vi "parse rest of message.vi"(5 "timeout/kb ms (1)":i32=1, 7 "continuation timeout ms (2000)":i32=2000, 8 "error in":errorcluster, 10 "mask(1)+length(7)":u8, 11 "lvlibretls connection in":refnum<data-value>) -> (0 "error out":errorcluster, 3 "unmasked data":string)   [LabVIEW 2016, in "websocket core.lvlib"]
uses:
  websocket core.lvlib
  lvlibtls/socket connection/lvlibretls connection.lvclass
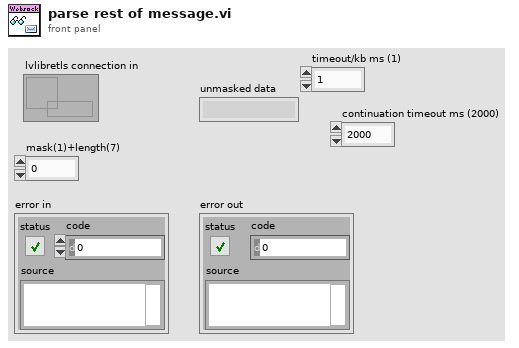
[diagram p1: front panel]
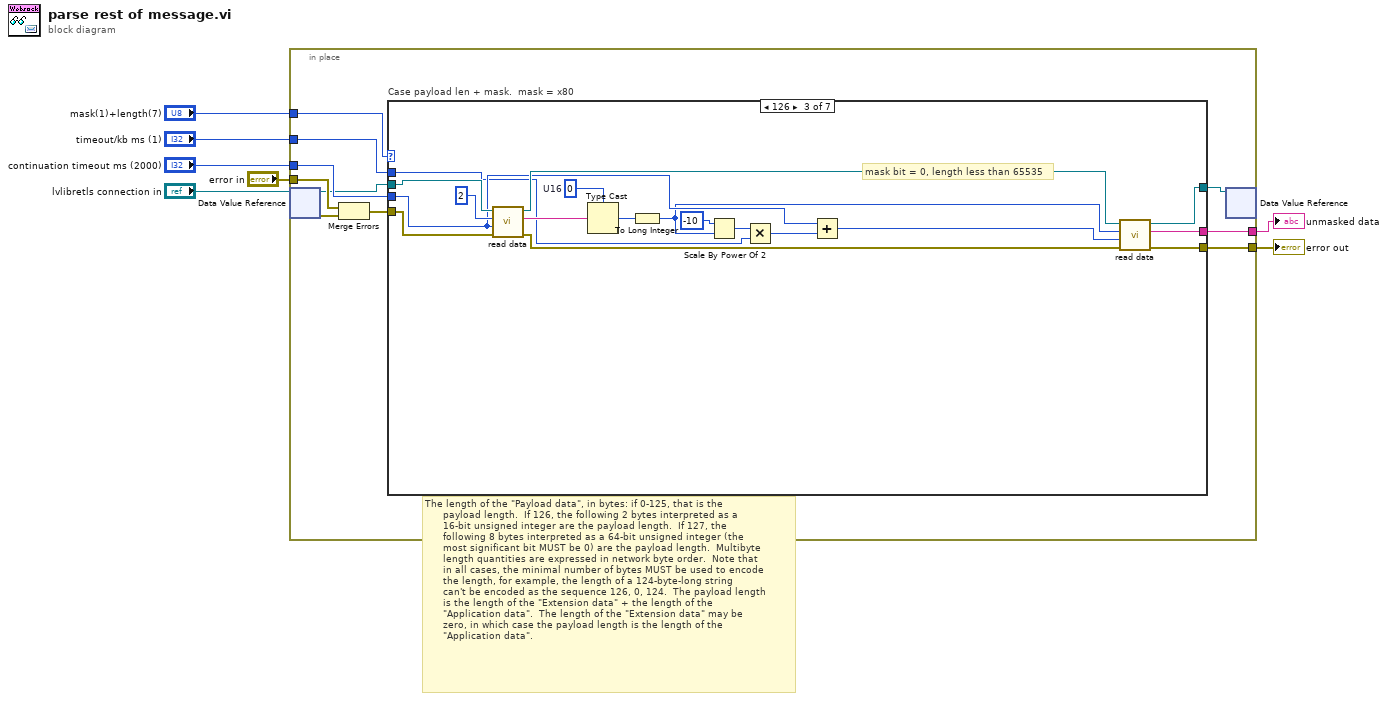
[diagram p0: block diagram]
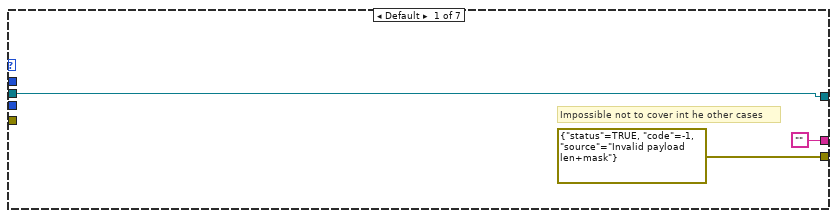
[diagram p2: hidden frame]
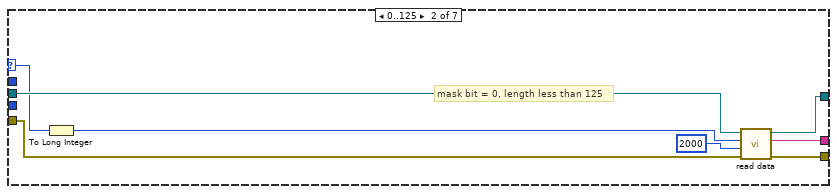
[diagram p3: hidden frame]
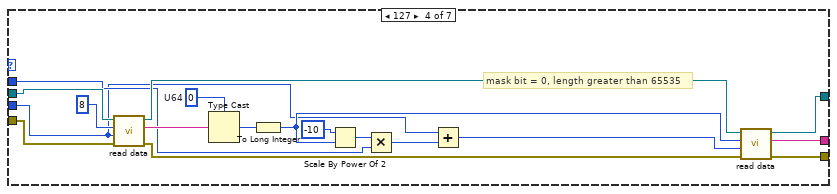
[diagram p4: hidden frame]
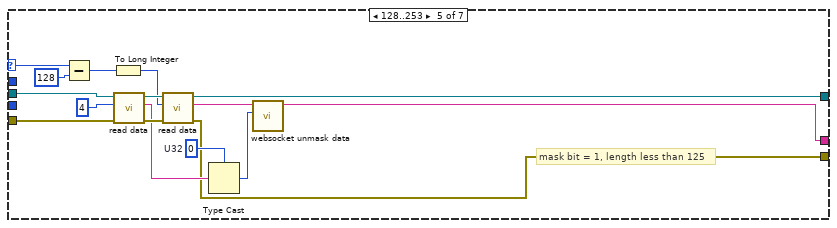
[diagram p5: hidden frame]
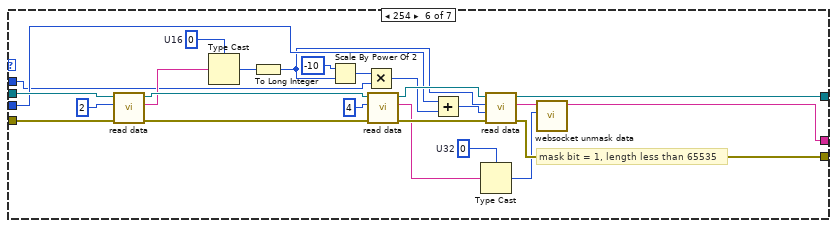
[diagram p6: hidden frame]
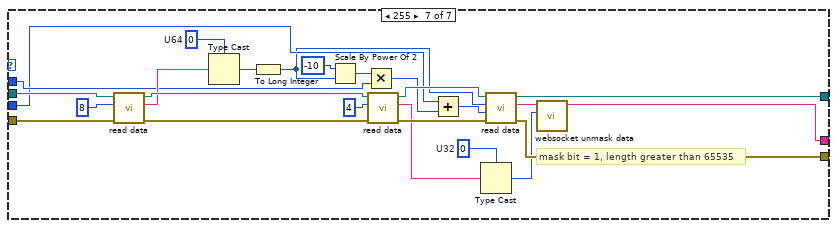
[diagram p7: hidden frame]
diagram:
  n1 = in-place {
    in-place-border: [w17] -> w7
    in-place-border: [w16] -> w6
    in-place-border: "mask(1)+length(7)" -> [w15]
    in-place-border: "error in" -> [w14]
    in-place-border: "continuation timeout ms (2000)" -> [w13]
    in-place-border: "timeout/kb ms (1)" -> [w12]
    # "The length of the \"Payload data\", in bytes: if 0-125, that is the\n      payload length.  If 126, the following 2 bytes interpreted as a\n      16-bit unsigned integer are the payload length.  If 127, the\n      following 8 bytes interpreted as a 64-bit unsigned integer (the\n      most significant bit MUST be 0) are the payload length.  Multibyte\n      length quantities are expressed in network byte order.  Note that\n      in all cases, the minimal number of bytes MUST be used to encode\n      the length, for example, the length of a 124-byte-long string\n      can't be encoded as the sequence 126, 0, 124.  The payload length\n      is the length of the \"Extension data\" + the length of the\n      \"Application data\".  The length of the \"Extension data\" may be\n      zero, in which case the payload length is the length of the\n      \"Application data\"."
    n2 = in-place-dvr #1("lvlibretls connection in") -> (w11:refnum<class "lvlibretls connection.lvclass">, w8:errorcluster)
    n3 = Merge Errors(w14, w8) -> (w9:errorcluster)
    n4 = case "Case payload len + mask.  mask = x80" shown="126" w15 {
      selector: w15 -> [_ w27 _ _ w79 _ _]
      tunnel: ["" w24 w39 w57 w68 w90 w115] -> w17
      tunnel: w11 -> [w18 w28 w46 w64 w80 w105 w130]
      tunnel: [errorcluster {"status"=TRUE, "code"=-1, "source"="Invalid payload len+mask"} ("error out") w23 w38 w56 w66 w94 w120] -> w16
      tunnel: w9 -> [_ w22 w37 w55 w70 w91 w116]
      tunnel: w13 -> [_ _ w36 w48 _ w85 w109]
      tunnel: w12 -> [_ _ w32 w49 _ w84 w110]
      tunnel: [w18 w21 w29 w47 w65 w81 w106] -> w10
      frame Default {
        # "Impossible not to cover int he other cases"
      }
      frame 0..125 {
        # "mask bit = 0, length less than 125"
        n5 = To Long Integer(number=w27) -> (32bit integer=w25:i32)
        n6 = call "read data.vi"("error in"=w22, "timeout"=2000 ("timeout ms (25000)"), "max size"=w25, "lvlibretls connection in"=w28) -> ("error out"=w23:errorcluster, "data"=w24:string, "lvlibretls connection out"=w21:refnum<class "lvlibretls connection.lvclass">)  [unwired: 5 in]
      }
      frame 126 {
        w40 = u16 0  # U16
        # "mask bit = 0, length less than 65535"
        n7 = call "read data.vi"("error in"=w37, "timeout"=w36, "max size"=2 ("bytes to read"), "lvlibretls connection in"=w46) -> ("error out"=w43:errorcluster, "data"=w42:string, "lvlibretls connection out"=w44:refnum<class "lvlibretls connection.lvclass">)  [unwired: 5 in]
        n8 = Type Cast(type=w40, x=w42) -> (*(type *) &x=w41:u16)
        n9 = To Long Integer(number=w41) -> (32bit integer=w35:i32)
        n10 = Scale By Power Of 2(n=i16 -10, x=w35) -> (x*2^n=w33:i32)
        n11 = Multiply(x=w33, y=w32) -> (x*y=w31:i32)
        n12 = Add(x=w36, y=w31) -> (x+y=w30:i32)
        n13 = call "read data.vi"("error in"=w43, "timeout"=w30, "max size"=w35, "lvlibretls connection in"=w44) -> ("error out"=w38:errorcluster, "data"=w39:string, "lvlibretls connection out"=w29:refnum<class "lvlibretls connection.lvclass">)  [unwired: 5 in]
      }
      frame 127 {
        w58 = u64 0  # U64
        # "mask bit = 0, length greater than 65535"
        n14 = call "read data.vi"("error in"=w55, "timeout"=w48, "max size"=8 ("bytes to read"), "lvlibretls connection in"=w64) -> ("error out"=w61:errorcluster, "data"=w60:string, "lvlibretls connection out"=w62:refnum<class "lvlibretls connection.lvclass">)  [unwired: 5 in]
        n15 = Type Cast(type=w58, x=w60) -> (*(type *) &x=w59:u64)
        n16 = To Long Integer(number=w59) -> (32bit integer=w51:i32)
        n17 = Scale By Power Of 2(n=i16 -10, x=w51) -> (x*2^n=w53:i32)
        n18 = Multiply(x=w53, y=w49) -> (x*y=w52:i32)
        n19 = Add(x=w48, y=w52) -> (x+y=w50:i32)
        n20 = call "read data.vi"("error in"=w61, "timeout"=w50, "max size"=w51, "lvlibretls connection in"=w62) -> ("error out"=w56:errorcluster, "data"=w57:string, "lvlibretls connection out"=w47:refnum<class "lvlibretls connection.lvclass">)  [unwired: 5 in]
      }
      frame 128..253 {
        w71 = u32 0  # U32
        # "mask bit = 1, length less than 125"
        n21 = Subtract(x=w79, y=u8 128) -> (x-y=w74:u8)
        n22 = To Long Integer(number=w74) -> (32bit integer=w73:i32)
        n23 = call "read data.vi"("error in"=w70, "max size"=4 ("bytes to read"), "lvlibretls connection in"=w80) -> ("error out"=w75:errorcluster, "data"=w72:string, "lvlibretls connection out"=w76:refnum<class "lvlibretls connection.lvclass">)  [unwired: 6 in]
        n24 = call "read data.vi"("error in"=w75, "max size"=w73, "lvlibretls connection in"=w76) -> ("error out"=w66:errorcluster, "data"=w69:string, "lvlibretls connection out"=w65:refnum<class "lvlibretls connection.lvclass">)  [unwired: 6 in]
        n25 = Type Cast(type=w71, x=w72) -> (*(type *) &x=w67:u32)
        n26 = call "websocket unmask data.vi"("mask key"=w67, "masked data"=w69) -> ("unmasked data"=w68:string)  [unwired: 9 in]
      }
      frame 254 {
        w92 = u32 0  # U32
        w99 = u16 0  # U16
        # "mask bit = 1, length less than 65535"
        n27 = call "read data.vi"("error in"=w91, "max size"=2 ("bytes to read"), "lvlibretls connection in"=w105) -> ("error out"=w102:errorcluster, "data"=w96:string, "lvlibretls connection out"=w103:refnum<class "lvlibretls connection.lvclass">)  [unwired: 6 in]
        n28 = Type Cast(type=w99, x=w96) -> (*(type *) &x=w100:u16)
        n29 = To Long Integer(number=w100) -> (32bit integer=w82:i32)
        n30 = Scale By Power Of 2(n=i16 -10, x=w82) -> (x*2^n=w87:i32)
        n31 = Multiply(x=w87, y=w84) -> (x*y=w86:i32)
        n32 = call "read data.vi"("error in"=w102, "max size"=4 ("bytes to read"), "lvlibretls connection in"=w103) -> ("error out"=w97:errorcluster, "data"=w93:string, "lvlibretls connection out"=w98:refnum<class "lvlibretls connection.lvclass">)  [unwired: 6 in]
        n33 = Add(x=w85, y=w86) -> (x+y=w83:i32)
        n34 = Type Cast(type=w92, x=w93) -> (*(type *) &x=w89:u32)
        n35 = call "read data.vi"("error in"=w97, "timeout"=w83, "max size"=w82, "lvlibretls connection in"=w98) -> ("error out"=w94:errorcluster, "data"=w95:string, "lvlibretls connection out"=w81:refnum<class "lvlibretls connection.lvclass">)  [unwired: 5 in]
        n36 = call "websocket unmask data.vi"("mask key"=w89, "masked data"=w95) -> ("unmasked data"=w90:string)  [unwired: 9 in]
      }
      frame 255 {
        w117 = u32 0  # U32
        w124 = u64 0  # U64
        # "mask bit = 1, length greater than 65535"
        n37 = call "read data.vi"("error in"=w116, "max size"=8 ("bytes to read"), "lvlibretls connection in"=w130) -> ("error out"=w127:errorcluster, "data"=w121:string, "lvlibretls connection out"=w128:refnum<class "lvlibretls connection.lvclass">)  [unwired: 6 in]
        n38 = Type Cast(type=w124, x=w121) -> (*(type *) &x=w125:u64)
        n39 = To Long Integer(number=w125) -> (32bit integer=w108:i32)
        n40 = Scale By Power Of 2(n=i16 -10, x=w108) -> (x*2^n=w112:i32)
        n41 = Multiply(x=w112, y=w110) -> (x*y=w111:i32)
        n42 = call "read data.vi"("error in"=w127, "max size"=4 ("bytes to read"), "lvlibretls connection in"=w128) -> ("error out"=w122:errorcluster, "data"=w118:string, "lvlibretls connection out"=w123:refnum<class "lvlibretls connection.lvclass">)  [unwired: 6 in]
        n43 = Add(x=w109, y=w111) -> (x+y=w107:i32)
        n44 = Type Cast(type=w117, x=w118) -> (*(type *) &x=w114:u32)
        n45 = call "read data.vi"("error in"=w122, "timeout"=w107, "max size"=w108, "lvlibretls connection in"=w123) -> ("error out"=w120:errorcluster, "data"=w119:string, "lvlibretls connection out"=w106:refnum<class "lvlibretls connection.lvclass">)  [unwired: 5 in]
        n46 = call "websocket unmask data.vi"("mask key"=w114, "masked data"=w119) -> ("unmasked data"=w115:string)  [unwired: 9 in]
      }
    }
    n47 = in-place-dvr #1(w10) -> ()  [unwired: 2 out]
  }
  "unmasked data" <- w7
  "error out" <- w6
